vi "A&N Recorder v4.0.vi"() -> ()   [LabVIEW 2016]
uses:
  <vilib>/sound2/lvsound2.llb/Sound File Refnum.ctl
  <vilib>/Analysis/3filter.llb/Filter Passband Type.ctl
  <vilib>/sound2/lvsound2.llb/Sound Data Format.ctl
  <vilib>/DAQmx/write.llb/DAQmx Write (Digital Bool 1Line 1Point).vi
  <vilib>/DAQmx/read.llb/DAQmx Read (Analog 1D Wfm NChan NSamp).vi
  <vilib>/DAQmx/miscellaneous.llb/DAQmx Fill In Error Info.vi
  <vilib>/Waveform/WDTOps.llb/WDT Index Channel DBL.vi
  Instance           7 25Saved   Detect&Record_014 .vi
  A&N Recorder v2.0/filename.vi
  <vilib>/sound2/lvsound2.llb/Sound File Write Open.vi
  <vilib>/sound2/lvsound2.llb/Sound File Write (DBL).vi
  Instance           1 25Saved   Detect&Record_014 .vi
  Instance           3 25Saved   Detect&Record_014 .vi
  <vilib>/Analysis/3filter.llb/Butterworth Filter (DBL).vi
  Instance           4 25Saved   Detect&Record_014 .vi
  Instance           5 25Saved   Detect&Record_014 .vi
  Instance           6 25Saved   Detect&Record_014 .vi
  <resource>/objmgr/daqmx.rc
  <vilib>/Analysis/NI_AALBase.lvlib
  <vilib>/DAQmx/read.llb/DAQmx Read (Digital Bool 1Line 1Point).vi
  <vilib>/Utility/error.llb/DialogType.ctl
panel:
  out "Data to Sent to Matlab":string="D:\\Dropbox\\LR73RY133\\2017-12-20\\LR73RY133_3596640997_2017_12_20_13_56_36.836.stm"
  in  "Port":u16=2057 min=1025 step=1
  in  "IP-Addresse":string="localhost" caption="Server IP Address"
  out "MATLAB ACK":bool
  out "File Ready":bool
  out "Cycles":i32
  out "DIO Heartbeat":bool=TRUE
  out "File Ready ONS":bool=TRUE
  in  "Spect Gain":i32=10
  in  "Gain 1":dbl=4.0
  in  "Offset 1":dbl=8.0
  in  "Low Cutoff (Hz)":dbl=300.0
  in  "High Cutoff (Hz)":dbl=15000.0
  out "Detect ONS":bool=TRUE
  out "Filename":string="LO58_3602250151_2018_02_23_12_02_31.268.wav"
  in  "Gain 2":dbl=3.0
  in  "Offset 2":dbl=5.0
  in  "Gain 3":dbl=3.0
  in  "Offset 3":dbl=1.0
  in  "Offset 4":dbl=-3.0
  in  "Gain 4":dbl=3.0
  in  "Gain 5":dbl=3.0
  in  "Offset 5":dbl=-7.0
  out "Waveform Chart":dbl[][](graph)
  out "sound file refnum out":T1
  out "Intensity Chart":dbl[][](graph)
  in  "#sw":bool=TRUE
  out "Song Detected":bool
  out "refnum out":refnum<file>
  out "refnum out WAV":refnum<file>
  in  "Mode Tab":T2(tab)
  out "Song Detection Vector":bool[](array[boolean])
  in  "Dectect window":i32=15
  out "Songs/Hour":u32(graph)=67
  in  "Song Detector":bool=TRUE
  in  "High Freq. Noise":dbl=350.0
  in  "Low Freq. Noise":dbl=50.0
  in  "High Freq. Song":dbl=7000.0
  in  "Low Freq. Song":dbl=2500.0
  in  "# Crossing per Samples\nSong Completed (OFF)":dbl
  in  "# Crossing per Samples\nSong Detected (ON)":dbl=4.0
  out "Current Ratio":dbl=0.03405842478239507 format="%#_3g"
  in  "Ratio Threshold":dbl=10.0
  out "SampQuant.SampPerChan":dbl=4410.0
  out "SampClk.Rate":dbl=44150.11037527594
  in  "Bird Birthday":timestamp=timestamp(3472056673.78125 s since 1904-01-01) format="%<%x>T"
  out "Bird Age":u32=411
  out "STM Open":bool
  in  "Save WAV":bool=TRUE
  in  "Save DAT":bool
  out "DAT Open":bool
  out "WAV Open":bool
  in  "File Prefix":string="LO58"
  in  "Current Record Index":dbl=14565.0
  in  "Path":path=path "D:/Dropbox/LO58"
  out "Append Path":path=path "D:/Dropbox/LO58/2018-02-23/LO58_3602250151_2018_02_23_12_02_31.268.wav"
  in  "Force Recording":bool
  out "#songs":u32=1
  out "Spontaneous Block Trigger":bool
  in  "Force Spont\nBlock":bool
  in  "Spont Block\nLength (min)":i32=1
  in  "Capture\nSpontaneous\nActivity":bool
  out "Current\nMinute":i32=2
  in  "Save STM":bool
  in  "STOP":bool
  # "Data Channels"
  # "Sound"
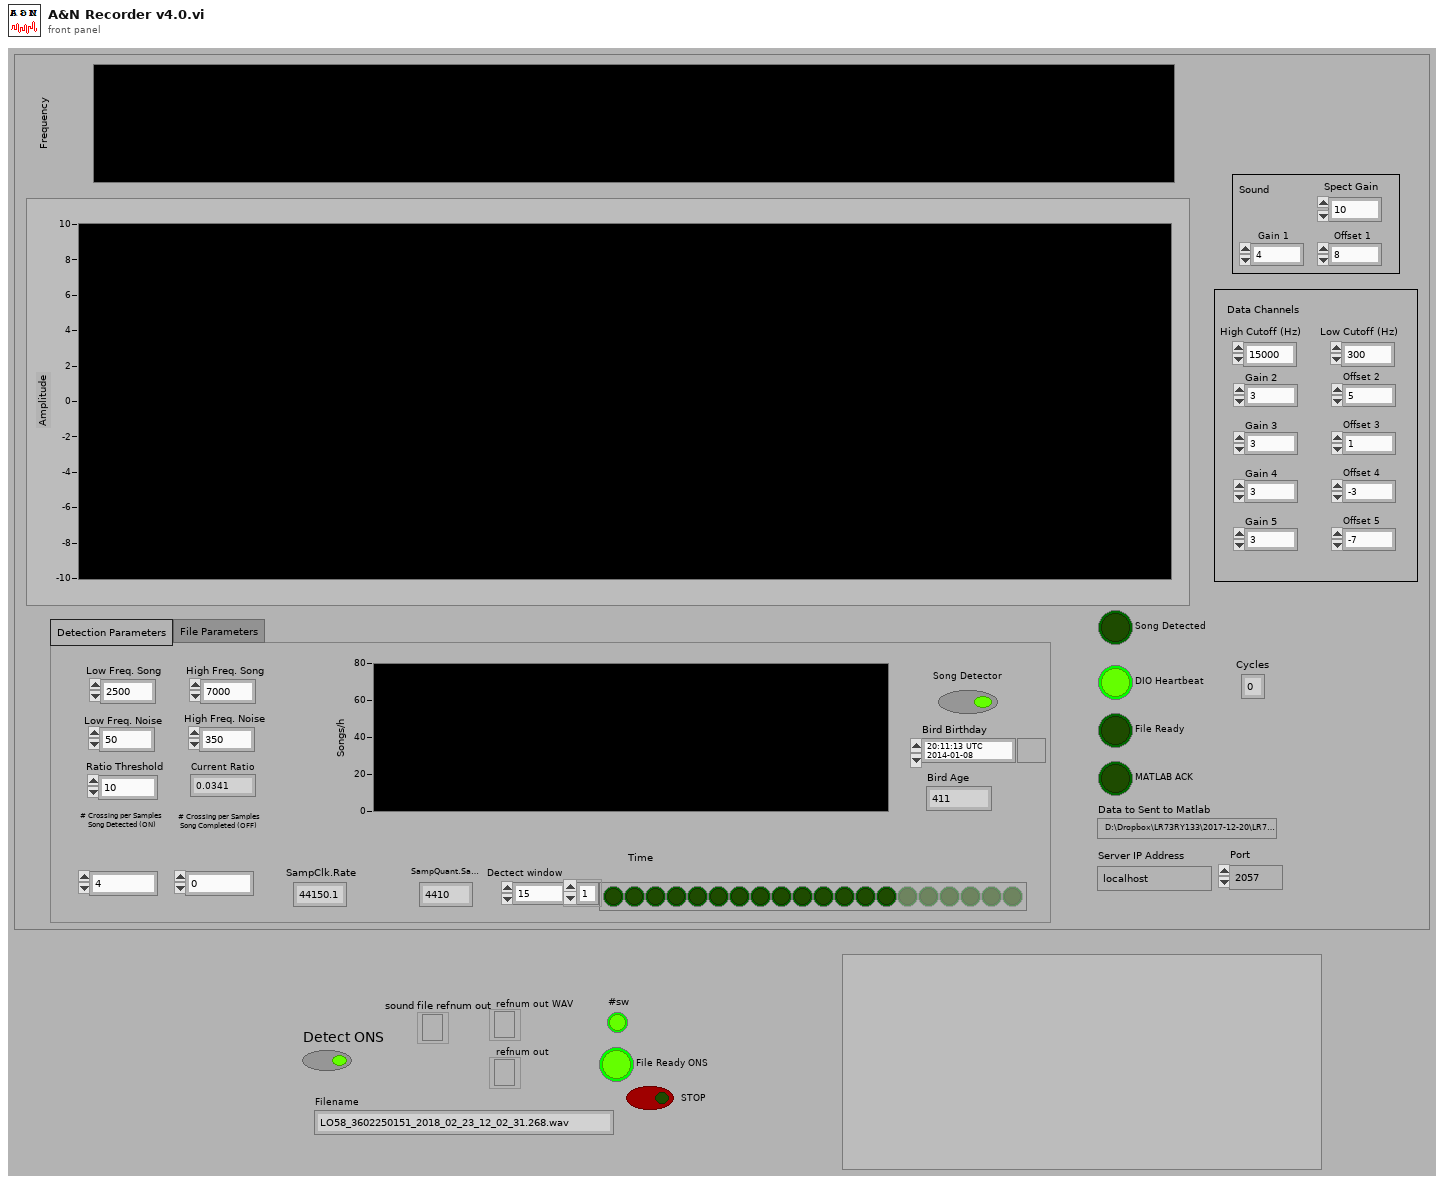
[diagram p1: front panel]
types:
  T1 = typedef "Sound File Refnum.ctl" = refnum<file>
  T2 = enum32{"Detection Parameters", "File Parameters"}
  T3 = cluster{"sound quality":enum16{"mono", "stereo"}, "bits per sample":enum16{"8 bit", "16 bit"}, "rate":u32}
  T4 = typedef "Sound Data Format.ctl" = cluster{"sample rate (S/s)":dbl, "number of channels":i32, "bits per sample":i32}
  T5 = enum16{"open", "replace", "create", "open or create", "replace or create", "replace or create with confirmation"}
  T6 = typedef "LVDateTimeRec.ctl" = cluster{"fractional second":dbl, "second":i32, "minute":i32, "hour":i32, "day of month":i32, "month":i32, "year":i32, "day of week":i32, "day of year":i32, "DST":i32}
  T7 = typedef "NI_AALBase.lvlib/Filter Passband Type.ctl" = enum32{"Lowpass", "Highpass", "Bandpass", "Bandstop"}
  T8 = cluster{"[0]":dbl, "[1]":dbl, "[2]":dbl, "[3]":dbl, "[4]":dbl, "[5]":dbl, "[6]":dbl, "[7]":dbl, "[8]":dbl, "[9]":dbl}
  T9 = typedef "DialogType.ctl" = u16
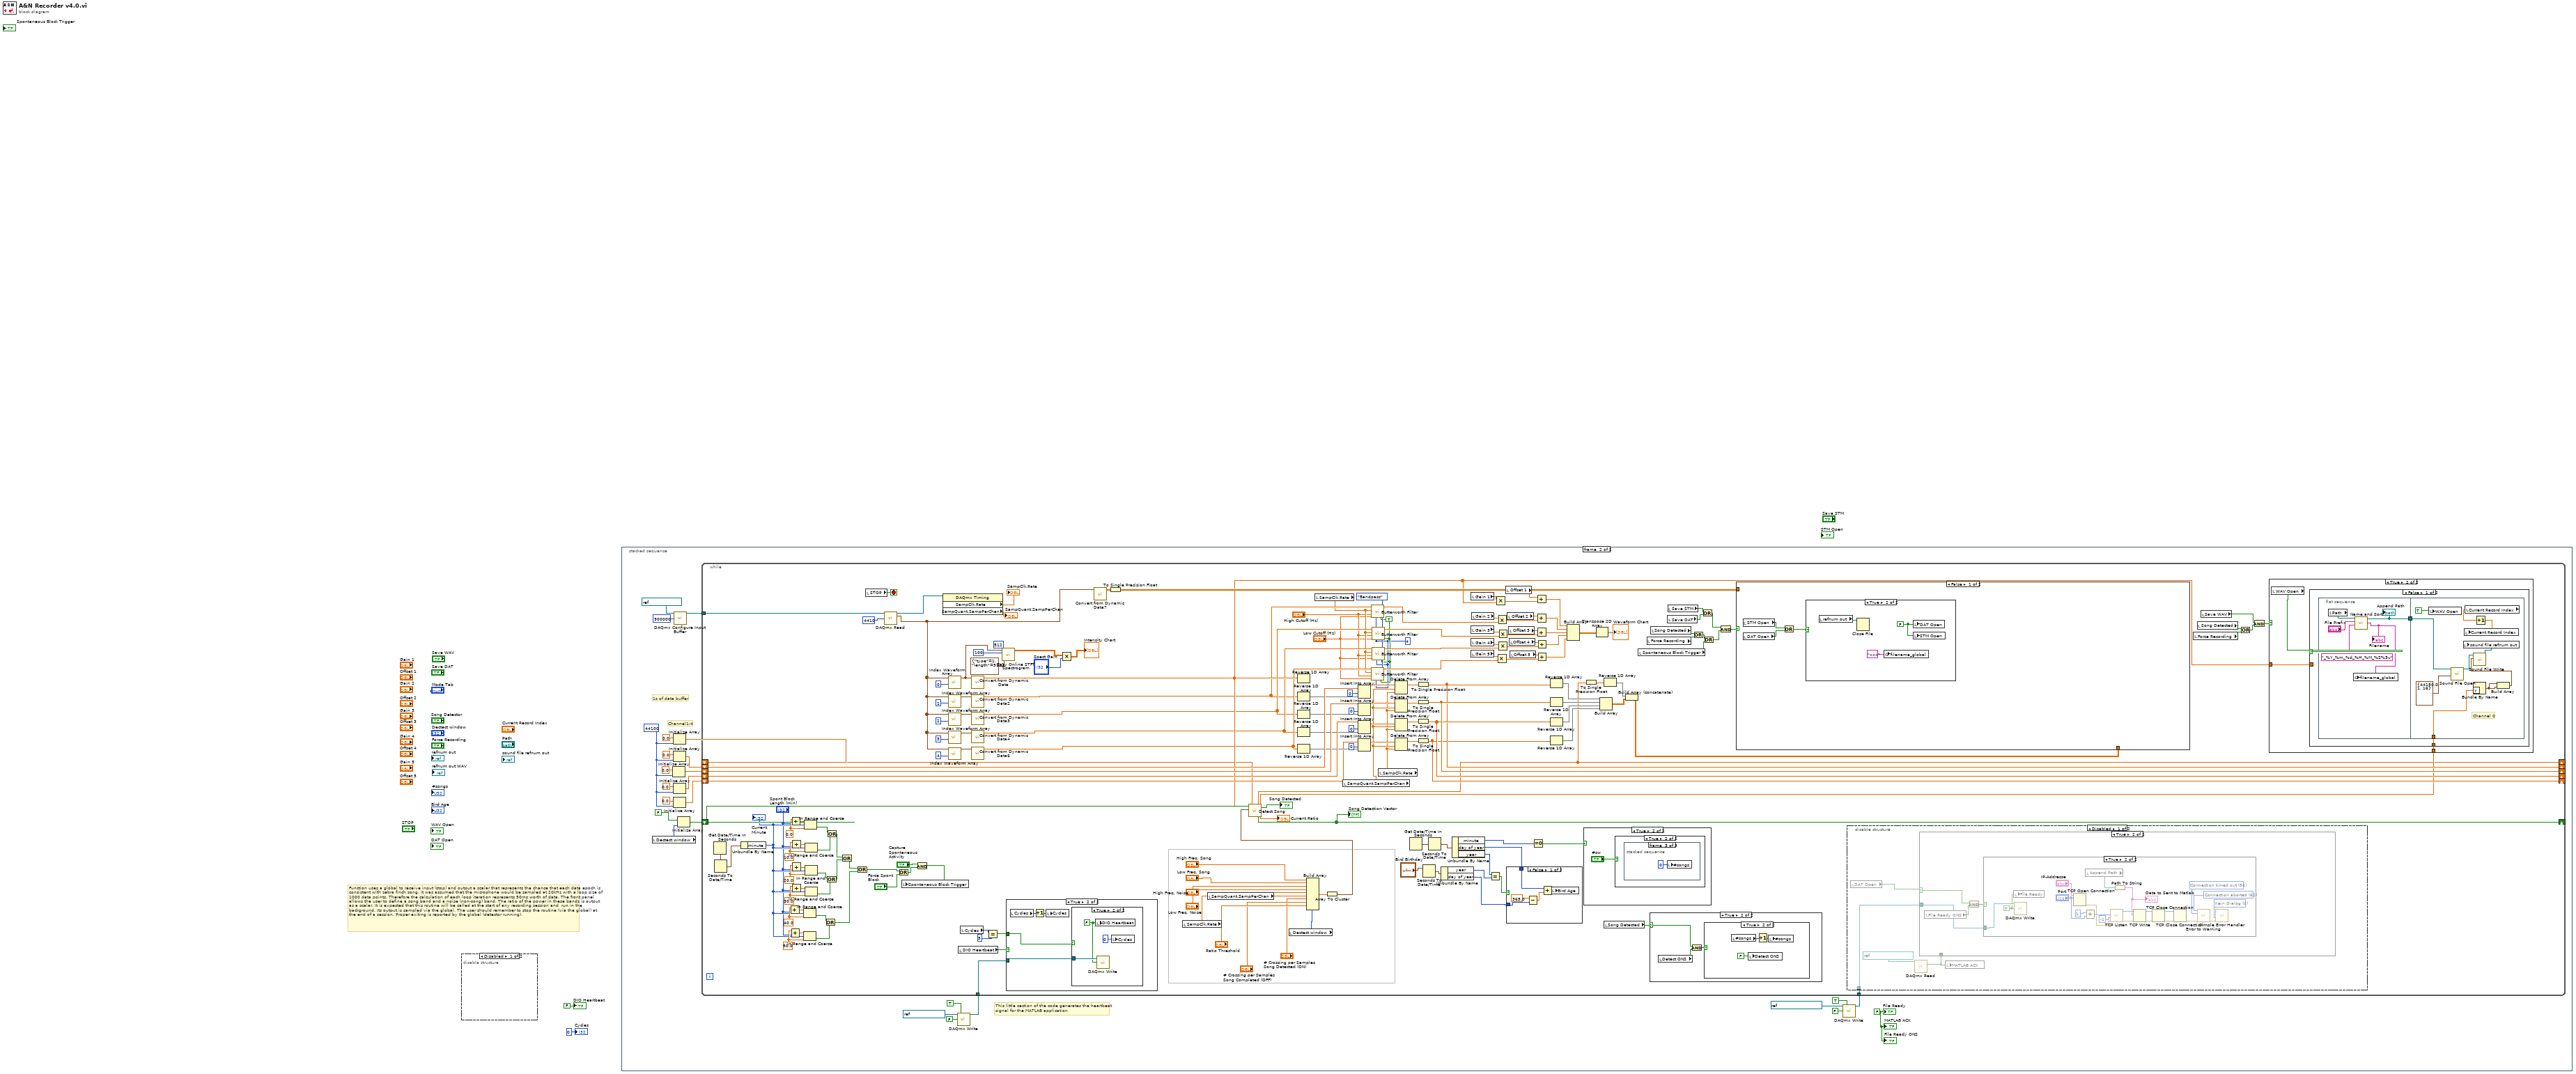
[diagram p0: block diagram]
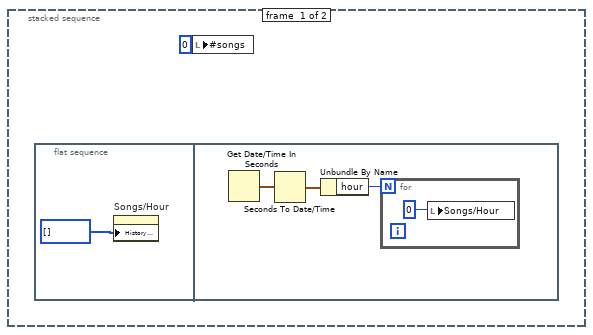
[diagram p3: hidden frame]
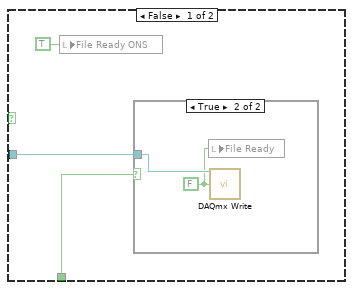
[diagram p4: hidden frame]
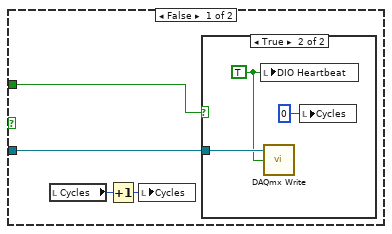
[diagram p8: hidden frame]
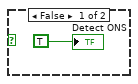
[diagram p11: hidden frame]
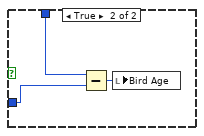
[diagram p13: hidden frame]
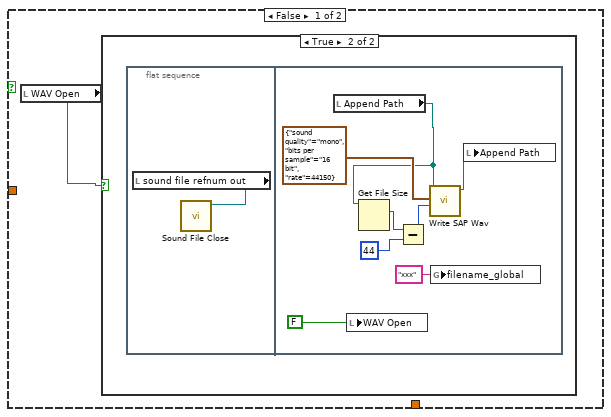
[diagram p14: hidden frame]
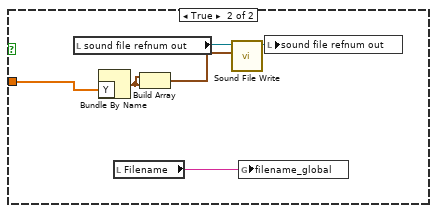
[diagram p16: hidden frame]
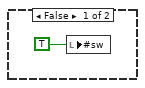
[diagram p17: hidden frame]
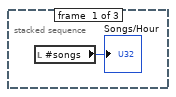
[diagram p19: hidden frame]
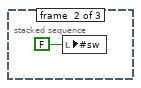
[diagram p20: hidden frame]
diagram:
  # "Function uses a global to receive input (stop) and output a scalar that represents the chance that each data epoch is consistent with zebra finch song. It was assumed that the microphone would be sampled at 20kHz with a loop size of 1000 data points. Therefore the calculation of each loop iteration represents 50ms worth of data. The front panel allows the user to define a song band and a noise (non-song) band. The ratio of the power in these bands is output as a scalar. It is expected that this routine will be called at the start of any recording session and  run in the background. Its output is sampled via the global. The user should remember to stop the routine (via the global) at the end of a session. Proper exiting is reported by the global (detector running)."
  n1 = disable-structure shown="Disabled" {
    frame Disabled {
    }
    frame Enabled {
    }
  }
  n2 = stacked-sequence {
    frame #0 {
      n3 = flat-sequence {
        frame #0 {
          n4 = property on="Songs/Hour" class="WFChart (strict)"("History Data"=u32[] []) -> ()  [unwired: 2 in, 2 out]
        }
        frame #1 {
          n5 = Get Date/Time In Seconds() -> (seconds since 1Jan1904=w6:timestamp)
          n6 = Seconds To Date/Time(time stamp (now)=w6) -> (date time rec=w7:T6)  [unwired: 1 out]
          n7 = Unbundle By Name(w7) -> ("hour"=w5:i32)
          n8 = for {
            N: w5 -> [_]
            n9 = local write "Songs/Hour"(0 ("element")) -> ()
          }
        }
      }
      n10 = local write "#songs"(u32 0 ("#songs")) -> ()
    }
    frame #1 {
      w9 = FALSE ("File Ready")
      w18 = 44100 ("dimension size")
      # "This little section of the code generates the heartbeat\nsignal for the MATLAB application"
      # "1s of data buffer"
      # "Channel1-4"
      n11 = local read "Dectect window"() -> (w24:i32)
      n12 = Initialize Array(sgl 0.0 ("element"), w18) -> (w26:sgl[])
      n13 = Initialize Array(sgl 0.0 ("element"), w18) -> (w25:sgl[])
      n14 = Initialize Array(sgl 0.0 ("element"), w18) -> (w23:sgl[])
      n15 = Initialize Array(sgl 0.0 ("element"), w18) -> (w28:sgl[])
      n16 = Initialize Array(sgl 0.0 ("element"), w18) -> (w27:sgl[])
      n17 = call <vilib>:"DAQmx Configure Input Buffer.vi"("task/channels in"=refnum<k21> "AN_Capture5", "buffer size (in samples per channel)"=u32 900000) -> ("task out"=w19:refnum<k21>)  [unwired: 1 in, 12 out]
      n18 = Initialize Array(FALSE, w24) -> (w33:bool[])
      n19 = call-poly <vilib>:"DAQmx Write.vi"("task/channels in"=refnum<k21> "AN_Heartbeat", "auto start"=TRUE, "data"=FALSE) -> ("task out"=w15:refnum<k21>)  [unwired: 1 in, 11 out]
      n20 = call-poly <vilib>:"DAQmx Write.vi"("task/channels in"=refnum<k21> "AN_SongFileReady", "auto start"=TRUE, "data"=FALSE) -> ("task out"=w10:refnum<k21>)  [unwired: 1 in, 11 out]
      n21 = while {
        shift-right: [w119] -> _
        shift-left: w33 -> [w138]
        shift-right: [w98] -> _
        shift-left: w28 -> [w135]
        shift-right: [w177] -> _
        shift-left: w27 -> [w206]
        shift-right: [w187] -> _
        shift-left: w26 -> [w204]
        shift-right: [w186] -> _
        shift-left: w25 -> [w202]
        shift-right: [w165] -> _
        shift-left: w23 -> [w161]
        tunnel: w19 -> [w143]
        tunnel: w15 -> [w40]
        tunnel: w10 -> [w35]
        stop <- w140 stop-if-true
        w51 = 50.0 ("upper limit")
        w52 = 40.0 ("upper limit")
        w62 = 30.0 ("upper limit")
        w61 = 20.0 ("upper limit")
        w60 = 10.0 ("upper limit")
        w59 = 0.0 ("upper limit")
        w82 = 4 ("order")
        w83 = TRUE ("init/cont (init:F)")
        w84 = Filter_Passband_Type."Bandpass" ("filter type")
        (unwired) 512 ("num of freq bins")
        n22 = Get Date/Time In Seconds() -> (seconds since 1Jan1904=w75:timestamp)
        n23 = Seconds To Date/Time(time stamp (now)=w75) -> (date time rec=w76:T6)  [unwired: 1 out]
        n24 = Unbundle By Name(w76) -> ("minute"=w48:i32)
        "Current\nMinute" <- w48
        n25 = Add(x=w52, y="Spont Block\nLength (min)") -> (x+y=w53:dbl)
        n26 = Add(x=w51, y="Spont Block\nLength (min)") -> (x+y=w54:dbl)
        n27 = Add(x=w59, y="Spont Block\nLength (min)") -> (x+y=w58:dbl)
        n28 = Add(x=w60, y="Spont Block\nLength (min)") -> (x+y=w57:dbl)
        n29 = Add(x=w61, y="Spont Block\nLength (min)") -> (x+y=w56:dbl)
        n30 = Add(x=w62, y="Spont Block\nLength (min)") -> (x+y=w55:dbl)
        n31 = In Range and Coerce(upper limit=w53, x=w48, lower limit=w52) -> (In Range?=w49:bool)  [unwired: 1 out]
        n32 = In Range and Coerce(upper limit=w54, x=w48, lower limit=w51) -> (In Range?=w50:bool)  [unwired: 1 out]
        n33 = In Range and Coerce(upper limit=w58, x=w48, lower limit=w59) -> (In Range?=w74:bool)  [unwired: 1 out]
        n34 = In Range and Coerce(upper limit=w57, x=w48, lower limit=w60) -> (In Range?=w73:bool)  [unwired: 1 out]
        n35 = In Range and Coerce(upper limit=w56, x=w48, lower limit=w61) -> (In Range?=w72:bool)  [unwired: 1 out]
        n36 = In Range and Coerce(upper limit=w55, x=w48, lower limit=w62) -> (In Range?=w71:bool)  [unwired: 1 out]
        n37 = Or(x=w49, y=w50) -> (x .or. y?=w46:bool)
        n38 = Or(x=w72, y=w71) -> (x .or. y?=w69:bool)
        n39 = Or(x=w74, y=w73) -> (x .or. y?=w70:bool)
        n40 = Or(x=w70, y=w69) -> (x .or. y?=w47:bool)
        n41 = Or(x=w47, y=w46) -> (x .or. y?=w45:bool)
        n42 = local read "STOP"() -> (w140:bool)
        n43 = call-poly <vilib>:"DAQmx Read.vi"("task/channels in"=w143, "number of samples per channel"=4410) -> ("task out"=w141:refnum<k21>, "data"=w142:waveform(dbl)[])  [unwired: 2 in, 10 out]
        n44 = Or(x=w45, y="Force Spont\nBlock") -> (x .or. y?=w65:bool)
        n45 = And(x="Capture\nSpontaneous\nActivity", y=w65) -> (x .and. y?=w64:bool)
        n46 = local write "Spontaneous Block Trigger"(w64) -> ()
        n47 = property class="DAQmx Timing"(reference=w141) -> ("SampClk.Rate"=→"SampClk.Rate":dbl, "SampQuant.SampPerChan"=→"SampQuant.SampPerChan":dbl)  [unwired: 1 in, 2 out]
        n48 = call-poly <vilib>:"Index Waveform Array.vi"("index"=0, "waveform array"=w142) -> ("waveform"=w139:waveform(dbl))  [unwired: 1 in, 8 out]
        n49 = call-poly <vilib>:"Index Waveform Array.vi"("index"=1, "waveform array"=w142) -> ("waveform"=w147:waveform(dbl))  [unwired: 1 in, 8 out]
        n50 = call-poly <vilib>:"Index Waveform Array.vi"("index"=2, "waveform array"=w142) -> ("waveform"=w152:waveform(dbl))  [unwired: 1 in, 8 out]
        n51 = call-poly <vilib>:"Index Waveform Array.vi"("index"=3, "waveform array"=w142) -> ("waveform"=w146:waveform(dbl))  [unwired: 1 in, 8 out]
        n52 = call-poly <vilib>:"Index Waveform Array.vi"("index"=4, "waveform array"=w142) -> ("waveform"=w145:waveform(dbl))  [unwired: 1 in, 8 out]
        n53 = local read "DIO Heartbeat"() -> (w39:bool)
        n54 = local read "Cycles"() -> (w38:i32)
        n55 = call "Convert from Dynamic Data"("Dynamic Data Type"=w139) -> ("Array"=w137:dbl[])  [unwired: 3 out]
        n56 = call "Convert from Dynamic Data2"("Dynamic Data Type"=w147) -> ("Array"=w86:dbl[])  [unwired: 3 out]
        n57 = call "Convert from Dynamic Data3"("Dynamic Data Type"=w152) -> ("Array"=w88:dbl[])  [unwired: 3 out]
        n58 = call "Convert from Dynamic Data4"("Dynamic Data Type"=w146) -> ("Array"=w90:dbl[])  [unwired: 3 out]
        n59 = call "Convert from Dynamic Data6"("Dynamic Data Type"=w145) -> ("Array"=w92:dbl[])  [unwired: 3 out]
        n60 = Equal?(x=w38, y=5) -> (x = y?=w36:bool)
        n61 = call <vilib>:"Easy Online STFT Spectrogram.vi"("window info"=cluster{"type":u16, "length":i32} {"type"=1, "length"=512}, "time interval"=100 ("frequency bins"), "signal in"=w139) -> ("Spec Block"=w94:dbl[][])  [unwired: 4 in, 4 out]
        n62 = case shown="True" w39 {
          tunnel: w40 -> [w249 w256]
          tunnel: w36 -> [w248 w253]
          frame False {
            n63 = local read "Cycles"() -> (w246:i32)
            n64 = Increment(x=w246) -> (x+1=w247:i32)
            n65 = local write "Cycles"(w247) -> ()
            n66 = case shown="True" w248 {
              tunnel: w249 -> [_ w252]
              frame False {
              }
              frame True {
                w251 = TRUE ("data")
                n67 = local write "DIO Heartbeat"(w251) -> ()
                n68 = call-poly <vilib>:"DAQmx Write.vi"("task/channels in"=w252, "data"=w251) -> ()  [unwired: 2 in, 12 out]
                n69 = local write "Cycles"(0 ("Cycles")) -> ()
              }
            }
          }
          frame True {
            n70 = local read "Cycles"() -> (w254:i32)
            n71 = Increment(x=w254) -> (x+1=w255:i32)
            n72 = local write "Cycles"(w255) -> ()
            n73 = case shown="True" w253 {
              tunnel: w256 -> [_ w259]
              frame False {
              }
              frame True {
                w258 = FALSE ("data")
                n74 = local write "DIO Heartbeat"(w258) -> ()
                n75 = call-poly <vilib>:"DAQmx Write.vi"("task/channels in"=w259, "data"=w258) -> ()  [unwired: 2 in, 12 out]
                n76 = local write "Cycles"(0 ("Cycles")) -> ()
              }
            }
          }
        }
        n77 = Multiply(x=w94, y="Spect Gain") -> (x*y=→"Intensity Chart":dbl[][])
        n78 = call "Convert from Dynamic Data7"("Dynamic Data Type"=w142) -> ("Array"=w151:dbl[][])  [unwired: 3 out]
        n79 = To Single Precision Float(number=w151) -> (single precision float=w150:sgl[][])
        n80 = local read "SampClk.Rate"() -> (w133:dbl)
        n81 = local read "SampQuant.SampPerChan"() -> (w132:dbl)
        n82 = local read "Dectect window"() -> (w123:i32)
        n83 = Reverse 1D Array(array=w137) -> ()  [unwired: 1 out]
        n84 = Reverse 1D Array(array=w86) -> (reversed array=w180:dbl[])
        n85 = Reverse 1D Array(array=w88) -> (reversed array=w179:dbl[])
        n86 = Reverse 1D Array(array=w90) -> (reversed array=w178:dbl[])
        n87 = Reverse 1D Array(array=w92) -> (reversed array=w166:dbl[])
        n88 = Build Array("High Freq. Song", "Low Freq. Song", "High Freq. Noise", "Low Freq. Noise", w132, w133, "# Crossing per Samples\nSong Detected (ON)", "# Crossing per Samples\nSong Completed (OFF)", "Ratio Threshold", w123) -> (w134:dbl[])
        n89 = local read "SampClk.Rate"() -> (w81:dbl)
        n90 = Array To Cluster(array=w134) -> (cluster=w124:T8)
        n91 = call "Detect Song.vi"("Audio Array"=w137, "Detect Parameters"=w124, "Dbl Shift In"=w135, "Bool Shift In"=w138) -> ("Dbl Shift Out"=w98:dbl[], "Bool Shift Out"=w119:bool[], "Buffered Audio To Save"=w121:dbl[], "Song Detect"=→"Song Detected":bool, "Current Ratio"=→"Current Ratio":dbl)  [unwired: 8 in, 3 out]
        "Song Detection Vector" <- w119
        n92 = local read "SampQuant.SampPerChan"() -> (w102:dbl)
        n93 = Insert Into Array(array=w206, index=0, new element=w180) -> (w183:sgl[])
        n94 = Insert Into Array(array=w204, index=0, new element=w179) -> (w182:sgl[])
        n95 = Insert Into Array(array=w202, index=0, new element=w178) -> (w181:sgl[])
        n96 = Insert Into Array(array=w161, index=0, new element=w166) -> (w167:sgl[])
        n97 = call-poly <vilib>:"Butterworth Filter.vi"("init/cont (init:F)"=w83, "order"=w82, "filter type"=w84, "low cutoff freq: fl"="Low Cutoff (Hz)", "high cutoff freq: fh"="High Cutoff (Hz)", "sampling freq: fs"=w81, "X"=w86) -> ("Filtered X"=w85:dbl[])  [unwired: 2 out]
        n98 = call-poly <vilib>:"Butterworth Filter.vi"("init/cont (init:F)"=w83, "order"=w82, "filter type"=w84, "low cutoff freq: fl"="Low Cutoff (Hz)", "high cutoff freq: fh"="High Cutoff (Hz)", "sampling freq: fs"=w81, "X"=w92) -> ("Filtered X"=w91:dbl[])  [unwired: 2 out]
        n99 = call-poly <vilib>:"Butterworth Filter.vi"("init/cont (init:F)"=w83, "order"=w82, "filter type"=w84, "low cutoff freq: fl"="Low Cutoff (Hz)", "high cutoff freq: fh"="High Cutoff (Hz)", "sampling freq: fs"=w81, "X"=w88) -> ("Filtered X"=w87:dbl[])  [unwired: 2 out]
        n100 = call-poly <vilib>:"Butterworth Filter.vi"("init/cont (init:F)"=w83, "order"=w82, "filter type"=w84, "low cutoff freq: fl"="Low Cutoff (Hz)", "high cutoff freq: fh"="High Cutoff (Hz)", "sampling freq: fs"=w81, "X"=w90) -> ("Filtered X"=w89:dbl[])  [unwired: 2 out]
        n101 = local read "SampClk.Rate"() -> (w101:dbl)
        n102 = Delete From Array(array=w183, length=w102, index=w101) -> (array with subset deleted=w184:sgl[])  [unwired: 1 out]
        n103 = Delete From Array(array=w182, length=w102, index=w101) -> (array with subset deleted=w195:sgl[])  [unwired: 1 out]
        n104 = Delete From Array(array=w181, length=w102, index=w101) -> (array with subset deleted=w189:sgl[])  [unwired: 1 out]
        n105 = Delete From Array(array=w167, length=w102, index=w101) -> (array with subset deleted=w168:sgl[])  [unwired: 1 out]
        n106 = Get Date/Time In Seconds() -> (seconds since 1Jan1904=w116:timestamp)
        n107 = To Single Precision Float(number=w184) -> (single precision float=w177:sgl[])
        n108 = To Single Precision Float(number=w195) -> (single precision float=w187:sgl[])
        n109 = To Single Precision Float(number=w189) -> (single precision float=w186:sgl[])
        n110 = To Single Precision Float(number=w168) -> (single precision float=w165:sgl[])
        n111 = Seconds To Date/Time(time stamp (now)="Bird Birthday") -> (date time rec=w118:T6)  [unwired: 1 out]
        n112 = Seconds To Date/Time(time stamp (now)=w116) -> (date time rec=w117:T6)  [unwired: 1 out]
        n113 = Unbundle By Name(w118) -> ("year"=w113:i32, "day of year"=w110:i32)
        n114 = Unbundle By Name(w117) -> ("minute"=w160:i32, "day of year"=w111:i32, "year"=w114:i32)
        n115 = local read "Gain 1"() -> (w199:dbl)
        n116 = local read "Gain 3"() -> (w192:dbl)
        n117 = local read "Gain 4"() -> (w176:dbl)
        n118 = local read "Gain 5"() -> (w163:dbl)
        n119 = local read "Gain 2"() -> (w198:dbl)
        n120 = Equal?(x=w114, y=w113) -> (x = y?=w112:bool)
        n121 = Multiply(x=w199, y=w137) -> (x*y=w201:dbl[])
        n122 = Multiply(x=w163, y=w91) -> (x*y=w149:dbl[])
        n123 = Multiply(x=w198, y=w85) -> (x*y=w197:dbl[])
        n124 = Multiply(x=w176, y=w89) -> (x*y=w191:dbl[])
        n125 = Multiply(x=w192, y=w87) -> (x*y=w194:dbl[])
        n126 = local read "Offset 1"() -> (w200:dbl)
        n127 = case shown="False" w112 {
          tunnel: w111 -> [w268 w274]
          tunnel: w110 -> [w270 w273]
          frame False {
            n128 = Subtract(x=365.0, y=w270) -> (x-y=w269:dbl)
            n129 = Add(x=w268, y=w269) -> (x+y=w267:dbl)
            n130 = local write "Bird Age"(w267) -> ()
          }
          frame True {
            n131 = Subtract(x=w274, y=w273) -> (x-y=w272:i32)
            n132 = local write "Bird Age"(w272) -> ()
          }
        }
        n133 = local read "Offset 2"() -> (w196:dbl)
        n134 = local read "Offset 3"() -> (w193:dbl)
        n135 = local read "Offset 4"() -> (w190:dbl)
        n136 = local read "Offset 5"() -> (w164:dbl)
        n137 = Equal To 0?(x=w160) -> (x = 0?=w159:bool)
        n138 = Add(x=w200, y=w201) -> (x+y=w174:dbl[])
        n139 = Add(x=w196, y=w197) -> (x+y=w173:dbl[])
        n140 = Add(x=w193, y=w194) -> (x+y=w172:dbl[])
        n141 = Add(x=w190, y=w191) -> (x+y=w171:dbl[])
        n142 = Add(x=w164, y=w149) -> (x+y=w162:dbl[])
        n143 = Reverse 1D Array(array=w177) -> (reversed array=w157:sgl[])
        n144 = Reverse 1D Array(array=w187) -> (reversed array=w156:sgl[])
        n145 = Reverse 1D Array(array=w186) -> (reversed array=w155:sgl[])
        n146 = Reverse 1D Array(array=w165) -> (reversed array=w154:sgl[])
        n147 = Build Array(w174, w173, w172, w171, w162) -> (w175:dbl[][])
        n148 = case shown="True" w159 {
          frame False {
            n149 = local write "#sw"(TRUE ("#sw")) -> ()
          }
          frame True {
            n150 = case shown="True" "#sw" {
              frame False {
              }
              frame True {
                n151 = stacked-sequence {
                  frame #0 {
                    n152 = local read "#songs"() -> (→"Songs/Hour":u32)
                  }
                  frame #1 {
                    n153 = local write "#sw"(FALSE ("#sw")) -> ()
                  }
                  frame #2 {
                    n154 = local write "#songs"(u32 0 ("#songs")) -> ()
                  }
                }
              }
            }
          }
        }
        n155 = To Single Precision Float(number=w98) -> (single precision float=w99:sgl[])
        n156 = Transpose 2D Array(2D array=w175) -> (transposed array=→"Waveform Chart":dbl[][])
        n157 = Build Array(w157, w156, w155, w154) -> (w153:sgl[][])
        n158 = Reverse 1D Array(array=w99) -> (reversed array=w100:sgl[])
        n159 = local read "Song Detected"() -> (w108:bool)
        n160 = Build Array (concatenate)(w100, w153) -> (w158:sgl[][])
        n161 = local read "Spontaneous Block Trigger"() -> (w66:bool)
        n162 = local read "Force Recording"() -> (w148:bool)
        n163 = case shown="True" w108 {
          selector: w108 -> [_ w261]
          frame False {
            "Detect ONS" <- TRUE
          }
          frame True {
            n164 = local read "Detect ONS"() -> (w262:bool)
            n165 = And(x=w261, y=w262) -> (x .and. y?=w263:bool)
            n166 = case shown="True" w263 {
              frame False {
              }
              frame True {
                n167 = local read "#songs"() -> (w265:u32)
                n168 = local write "Detect ONS"(FALSE ("Detect ONS")) -> ()
                n169 = Increment(x=w265) -> (x+1=w266:u32)
                n170 = local write "#songs"(w266) -> ()
              }
            }
          }
        }
        n171 = local read "Song Detected"() -> (w185:bool)
        n172 = local read "Save DAT"() -> (w43:bool)
        n173 = local read "Save STM"() -> (w41:bool)
        n174 = Or(x=w185, y=w148) -> (x .or. y?=w68:bool)
        n175 = Or(x=w41, y=w43) -> (x .or. y?=w42:bool)
        n176 = Or(x=w68, y=w66) -> (x .or. y?=w67:bool)
        n177 = And(x=w42, y=w67) -> (x .and. y?=w188:bool)
        n178 = case shown="False" w188 {
          tunnel: w158 -> [_ w326]
          tunnel: w150 -> [_ w325]
          frame False {
            n179 = local read "STM Open"() -> (w317:bool)
            n180 = local read "DAT Open"() -> (w316:bool)
            n181 = Or(x=w317, y=w316) -> (x .or. y?=w318:bool)
            n182 = case shown="True" w318 {
              frame False {
              }
              frame True {
                w319 = FALSE ("File Open")
                n183 = local read "refnum out"() -> (w321:refnum<file>)
                n184 = Close File(refnum=w321) -> ()  [unwired: 1 in, 2 out]
                n185 = global write "filename.vi" "filename_global"("xxx" ("wavefile_global_a7")) -> ()
                n186 = local write "DAT Open"(w319) -> ()
                n187 = local write "STM Open"(w319) -> ()
              }
            }
          }
          frame True {
            n188 = local read "DAT Open"() -> (w323:bool)
            n189 = local read "STM Open"() -> (w322:bool)
            n190 = Or(x=w322, y=w323) -> (x .or. y?=w324:bool)
            n191 = case shown="False" w324 {
              tunnel: w326 -> [w327 _]
              tunnel: w325 -> [_ w368]
              frame False {
                n192 = flat-sequence {
                  tunnel: [w334] -> w328
                  tunnel: w328 -> [w352]
                  tunnel: w327 -> [w351]
                  frame #0 {
                    n193 = local read "Spontaneous Block Trigger"() -> (w335:bool)
                    n194 = case shown="True" w335 {
                      tunnel: [w346 w347] -> w331
                      frame False {
                        n195 = local read "Path"() -> (w346:path)
                      }
                      frame True {
                        n196 = local read "Path"() -> (w349:path)
                        n197 = Build Path(base path=w349, name or relative path="Spon") -> (appended path=w347:path)
                      }
                    }
                    n198 = local read "File Prefix"() -> (w330:string)
                    n199 = local read "Save DAT"() -> (w333:bool)
                    n200 = case shown="True" w333 {
                      tunnel: [w340 w345] -> w334
                      tunnel: [w339 w344] -> w329
                      tunnel: w331 -> [w338 w343]
                      tunnel: w330 -> [w337 w342]
                      tunnel: "_%Y_%m_%d_%H_%M_%S%3u" ("time format string (%c)") -> [w336 w341]
                      frame False {
                        n201 = call "Name and Sort STM.vi"("Time Stamp Format"=w336, "Bird Name"=w337, "Root Folder"=w338) -> ("Filename"=w339:string, "Append Path"=w340:path)  [unwired: 2 in]
                      }
                      frame True {
                        n202 = call "Name and Sort DAT.vi"("Time Stamp Format"=w341, "Bird Name"=w342, "Root Folder"=w343) -> ("Filename"=w344:string, "Append Path"=w345:path)  [unwired: 2 out]
                      }
                    }
                    n203 = global write "filename.vi" "filename_global"(w329) -> ()
                    n204 = local write "Filename"(w329) -> ()
                  }
                  frame #1 {
                    n205 = local read "Current Record Index"() -> (w365:dbl)
                    n206 = Open/Create/Replace File(file path (use dialog)=w352, operation (0:open)=T5."replace or create") -> (refnum out=w356:refnum<file>, error out=w354:errorcluster)  [unwired: 1 in, 4 out]
                    n207 = Increment(x=w365) -> (x+1=w366:dbl)
                    n208 = Build Array(sgl 44150.0 ("element"), sgl 1000.0, sgl 5.0) -> (w360:sgl[])
                    n209 = local write "Current Record Index"(w366) -> ()
                    n210 = Write to Binary File(file (use dialog)=w356, data=w360, error in=w354, 5:FALSE ("prepend array or string size? (T)")) -> (refnum out=w353:refnum<file>, error out=w355:errorcluster)  [unwired: 1 in, 2 out]
                    n211 = Write to Binary File(file (use dialog)=w353, data=w351, error in=w355, 5:FALSE ("prepend array or string size? (T)")) -> (refnum out=w361:refnum<file>)  [unwired: 4 out]
                    n212 = local write "refnum out"(w361) -> ()
                    n213 = local write "DAT Open"(TRUE ("File Open")) -> ()
                  }
                }
              }
              frame True {
                n214 = local read "Filename"() -> (w367:string)
                n215 = local read "refnum out"() -> (w370:refnum<file>)
                n216 = global write "filename.vi" "filename_global"(w367) -> ()
                n217 = Write to Binary File(file (use dialog)=w370, data=w368, 5:FALSE ("prepend array or string size? (T)")) -> (refnum out=w371:refnum<file>)  [unwired: 1 in, 4 out]
                n218 = local write "refnum out"(w371) -> ()
              }
            }
          }
        }
        n219 = disable-structure shown="Disabled" {
          disable-tunnel: w35 -> [w215 _]
          frame Disabled {
            n220 = local read "DAT Open"() -> (w214:bool)
            n221 = call-poly <vilib>:"DAQmx Read.vi"("task/channels in"=refnum<k21> "AN_MATLAB_ACK") -> ("data"=w213:bool)  [unwired: 12 in, 2 out]
            n222 = case shown="True" w214 {
              selector: w214 -> [_ w222]
              tunnel: w215 -> [w217 w221]
              tunnel: w213 -> [w216 _]
              frame False {
                n223 = local write "File Ready ONS"(TRUE ("File Ready ONS")) -> ()
                n224 = case shown="True" w216 {
                  tunnel: w217 -> [_ w220]
                  frame False {
                  }
                  frame True {
                    w219 = FALSE ("data")
                    n225 = local write "File Ready"(w219) -> ()
                    n226 = call-poly <vilib>:"DAQmx Write.vi"("task/channels in"=w220, "data"=w219) -> ()  [unwired: 2 in, 12 out]
                  }
                }
              }
              frame True {
                n227 = local read "File Ready ONS"() -> (w223:bool)
                n228 = And(x=w222, y=w223) -> (x .and. y?=w224:bool)
                n229 = case shown="True" w224 {
                  tunnel: w221 -> [_ w245]
                  frame False {
                  }
                  frame True {
                    w243 = T9 0 items=["Kein Dialog", "OK-Meldung", "Dialog zum Fortsetzen oder Anhalten", "OK-Meldung + Warnungen", "Weiter/Stopp + Warnung"] ("type of dialog (OK msg:1)")
                    w239 = 56 items=["No Error", "Argument Error", "Memory Full", "Out of Zone", "End of File", "File Already Open", "Generic File IO Error", "File Not Found", "File Permission Error", "Disk Full", "Duplicate Path", "Too Many Files Open", "Not Enabled", "Resource File Not Found", "Cannot Add Resource", "Resource Not Found", "Image Not Found", "Image Memory Error", "Pen Does Not Exist", "Config Bad Type", "Config Token Not Found", "Config Parse Error", "Config Memory Error", "Bad External Code Format", "Bad External Code Offset", "External Code Not Present", "Null Window", "Destroy Window Mixup", "Null Menu", "Print Aborted", "Bad Print Record", "Print Driver Error", "Windows Error During Print", "Memory Error During Print", "Print Dialog Error", "Generic Print Error", "Invalid Device Refnum", "Device Not Found", "Device Parameter Error", "Device Unit Error", "Can't Open Device", "Device Call Aborted", "Generic Error", "Cancelled By User", "Object ID Too Low", "Object ID Too High", "Object Not In Heap", "Unknown Heap", "Bad DefProc ID", "DefProc Not In Table", "Message Out Of Range", "Null Method", "Unknown Message", "Manager Call Not Supported", "Bad address", "Connection In progress", "Connection timed out", "Connection is already in progress", "Network attribute not supported", "Network error", "Address in use", "System out of memory", "Connection aborted", "Connection refused", "Connection is not connected", "Connection is already connected", "Connection closed", "Initialize error (interapplication manager)", "Bad occurrence", "Wait on unbound occurrence handler", "Occurrence queue overflow", "Bad path", "Semaphore not signaled", "Unrecognized type (interapplication manager)"] ("2nd Error to Convert")
                    w238 = 62 items=["No Error", "Argument Error", "Memory Full", "Out of Zone", "End of File", "File Already Open", "Generic File IO Error", "File Not Found", "File Permission Error", "Disk Full", "Duplicate Path", "Too Many Files Open", "Not Enabled", "Resource File Not Found", "Cannot Add Resource", "Resource Not Found", "Image Not Found", "Image Memory Error", "Pen Does Not Exist", "Config Bad Type", "Config Token Not Found", "Config Parse Error", "Config Memory Error", "Bad External Code Format", "Bad External Code Offset", "External Code Not Present", "Null Window", "Destroy Window Mixup", "Null Menu", "Print Aborted", "Bad Print Record", "Print Driver Error", "Windows Error During Print", "Memory Error During Print", "Print Dialog Error", "Generic Print Error", "Invalid Device Refnum", "Device Not Found", "Device Parameter Error", "Device Unit Error", "Can't Open Device", "Device Call Aborted", "Generic Error", "Cancelled By User", "Object ID Too Low", "Object ID Too High", "Object Not In Heap", "Unknown Heap", "Bad DefProc ID", "DefProc Not In Table", "Message Out Of Range", "Null Method", "Unknown Message", "Manager Call Not Supported", "Bad address", "Connection In progress", "Connection timed out", "Connection is already in progress", "Network attribute not supported", "Network error", "Address in use", "System out of memory", "Connection aborted", "Connection refused", "Connection is not connected", "Connection is already connected", "Connection closed", "Initialize error (interapplication manager)", "Bad occurrence", "Wait on unbound occurrence handler", "Occurrence queue overflow", "Bad path", "Semaphore not signaled", "Unrecognized type (interapplication manager)"] ("1st Error to Convert")
                    w244 = TRUE ("data")
                    n230 = local write "File Ready"(w244) -> ()
                    n231 = call-poly <vilib>:"DAQmx Write.vi"("task/channels in"=w245, "data"=w244) -> ()  [unwired: 2 in, 12 out]
                    n232 = TCP Open Connection(address="IP-Addresse", remote port or service name="Port") -> (error out=w225:errorcluster)  [unwired: 3 in, 1 out]
                    n233 = Add(x=u16 1, y="Port") -> (x+y=w231:u16)
                    n234 = local read "Append Path"() -> (w227:path)
                    n235 = call <vilib>:"TCP Listen.vi"("error in (no error)"=w225, "timeout ms (wait forever: -1)"=-1, "port"=w231) -> ("error out"=w233:errorcluster, "connection ID"=w232:refnum<k5>)  [unwired: 4 in, 3 out]
                    n236 = Path To String(path=w227) -> (string=w226:string)
                    "Data to Sent to Matlab" <- w226
                    n237 = TCP Write(connection ID=w232, data in=w226, error in (no error)=w233) -> (connection ID out=w242:refnum<k5>, error out=w235:errorcluster)  [unwired: 1 in, 1 out]
                    n238 = TCP Close Connection(connection ID=w242, error in (no error)=w235) -> (connection ID out=w240:refnum<k5>, error out=w241:errorcluster)  [unwired: 1 in]
                    n239 = TCP Close Connection(connection ID=w240, error in (no error)=w241) -> (error out=w236:errorcluster)  [unwired: 1 in, 1 out]
                    n240 = call <vilib>:"Error to Warning.vi"("1st Error to Convert"=w238, "2nd Error to Convert"=w239, "error in"=w236) -> ("warning out"=w237:errorcluster)  [unwired: 12 in]
                    n241 = call <vilib>:"Simple Error Handler.vi"("type of dialog (OK msg:1)"=w243, "error in (no error)"=w237) -> ()  [unwired: 3 in, 5 out]
                  }
                }
              }
            }
            n242 = local write "MATLAB ACK"(w213) -> ()
          }
          frame Enabled {
          }
        }
        n243 = local read "Force Recording"() -> (w106:bool)
        n244 = local read "Song Detected"() -> (w104:bool)
        n245 = local read "Save WAV"() -> (w105:bool)
        n246 = Or(x=w104, y=w106) -> (x .or. y?=w107:bool)
        n247 = And(x=w105, y=w107) -> (x .and. y?=w103:bool)
        n248 = case shown="True" w103 {
          tunnel: w121 -> [_ w287]
          tunnel: w137 -> [_ w286]
          frame False {
            n249 = local read "WAV Open"() -> (w275:bool)
            n250 = case shown="True" w275 {
              frame False {
              }
              frame True {
                n251 = flat-sequence {
                  frame #0 {
                    n252 = local read "sound file refnum out"() -> (w276:T1)
                    n253 = call <vilib>:"Sound File Close.vi"("sound file refnum"=w276) -> ()  [unwired: 1 in, 10 out]
                  }
                  frame #1 {
                    n254 = local read "Append Path"() -> (w282:path)
                    n255 = local write "WAV Open"(FALSE ("File Open")) -> ()
                    n256 = Get File Size(file=w282) -> (size (in bytes)=w280:i64)  [unwired: 1 in, 2 out]
                    n257 = Subtract(x=w280, y=i64 44) -> (x-y=w281:i64)
                    n258 = call "Write SAP Wav.vi"("Audio Size ( bytes)"=w281, "input cluster"=T3 {"sound quality"=enum."mono", "bits per sample"=enum."16 bit", "rate"=44150}, "wave file path"=w282) -> ("wave file path out"=w283:path)  [unwired: 1 in, 7 out]
                    n259 = global write "filename.vi" "filename_global"("xxx" ("filename_global")) -> ()
                    n260 = local write "Append Path"(w283) -> ()
                  }
                }
              }
            }
          }
          frame True {
            n261 = local read "WAV Open"() -> (w285:bool)
            n262 = case shown="False" w285 {
              tunnel: w287 -> [w289 _]
              tunnel: w286 -> [_ w306]
              frame False {
                n263 = flat-sequence {
                  tunnel: [w291] -> w288
                  tunnel: w289 -> [w295]
                  tunnel: w288 -> [w297]
                  frame #0 {
                    n264 = local read "Path"() -> (w294:path)
                    n265 = call "Name and Sort.vi"("Time Stamp Format"="_%Y_%m_%d_%H_%M_%S%3u" ("time format string (%c)"), "Bird Name"="File Prefix", "Root Folder"=w294) -> ("Filename"=w290:string, "Append Path"=w291:path)  [unwired: 2 out]
                    "Append Path" <- w291
                    "Filename" <- w290
                    n266 = global write "filename.vi" "filename_global"(w290) -> ()
                  }
                  frame #1 {
                    # "Channel 0"
                    n267 = local write "WAV Open"(TRUE ("File Open")) -> ()
                    n268 = call-poly <vilib>:"Sound File Open.vi"("sound format"=T4 {"sample rate (S/s)"=44150.0, "number of channels"=1, "bits per sample"=16}, "path"=w297) -> ("sound file refnum"=w300:T1)  [unwired: 1 in, 8 out]
                    n269 = local read "Current Record Index"() -> (w303:dbl)
                    n270 = Bundle By Name("Y"=w295) -> (w298:waveform(dbl))  [unwired: 1 out]
                    n271 = Increment(x=w303) -> (x+1=w304:dbl)
                    n272 = local write "Current Record Index"(w304) -> ()
                    n273 = Build Array(w298, w298) -> (w299:waveform(dbl)[])
                    n274 = call-poly <vilib>:"Sound File Write.vi"("data"=w299, "sound file refnum"=w300) -> ("sound file refnum out"=w301:T1)  [unwired: 1 in, 8 out]
                    n275 = local write "sound file refnum out"(w301) -> ()
                  }
                }
              }
              frame True {
                n276 = local read "sound file refnum out"() -> (w310:T1)
                n277 = Bundle By Name("Y"=w306) -> (w308:waveform(dbl))  [unwired: 1 out]
                n278 = local read "Filename"() -> (w305:string)
                n279 = Build Array(w308, w308) -> (w307:waveform(dbl)[])
                n280 = call-poly <vilib>:"Sound File Write.vi"("data"=w307, "sound file refnum"=w310) -> ("sound file refnum out"=w309:T1)  [unwired: 1 in, 8 out]
                n281 = global write "filename.vi" "filename_global"(w305) -> ()
                n282 = local write "sound file refnum out"(w309) -> ()
              }
            }
          }
        }
      }
      "File Ready" <- w9
      "File Ready ONS" <- w9
      "MATLAB ACK" <- w9
    }
  }
  "DIO Heartbeat" <- FALSE ("DIO Heartbeat")
  "Cycles" <- 0 ("Cycles")
